vi "Script Edit Module Name.vi"(8 "error in":errorcluster, 10 "Library":refnum<class "Library.lvclass">, 11 "Project":refnum<class "Project.lvclass">) -> (0 "error out":errorcluster)   [LabVIEW 2020, in "Panther Dashboard.lvlib"]
uses:
  Panther Dashboard.lvlib
  Class/Library/Library.lvclass
  C:/GitClones/PantherDashboard/src/LabVIEW/Panther Dashboard/Class/LabVIEWItem/LabVIEWItem.lvclass
  Class/Project/Project.lvclass
  <vilib>/Utility/traverseref.llb/TRef TravTarget.ctl
  Class/Project/Project.lvclass/Project.ctl
  Class/LabVIEWItem/LabVIEWItem.lvclass/LabVIEWItem.ctl
  Class/Project/Read Main App Inst Ref.vi
  Class/LabVIEWItem/Read Item Path.vi
  <vilib>/Utility/traverseref.llb/VI Scripting - Traverse.lvlib
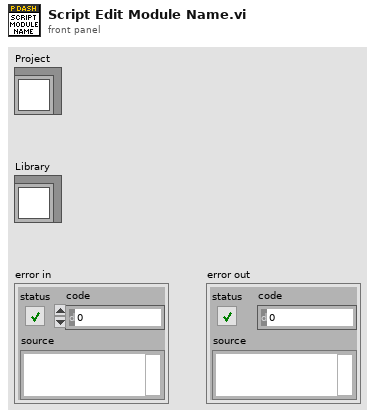
[diagram p1: front panel]
types:
  T1 = typedef "TRef TravTarget.ctl" = enum16{"FP", "BD", "Other"}
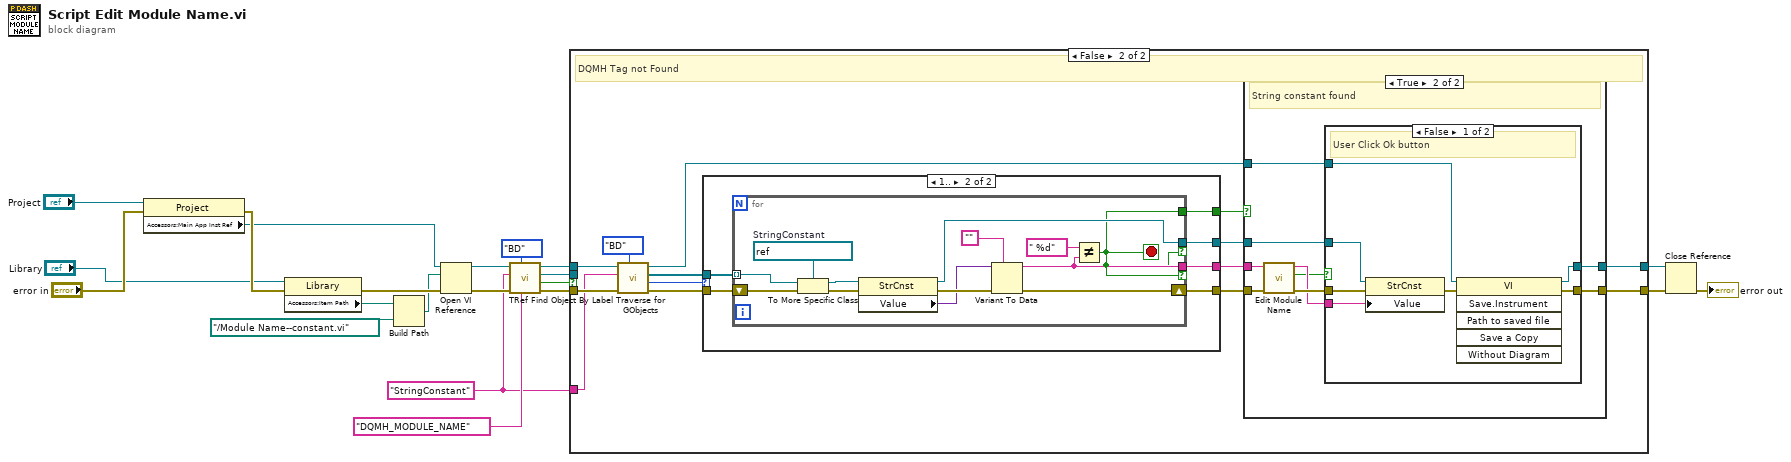
[diagram p0: block diagram]
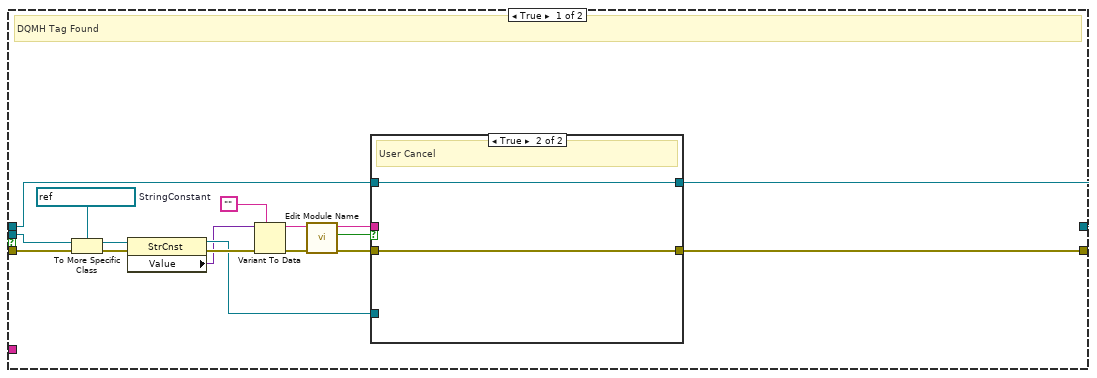
[diagram p2: hidden frame]
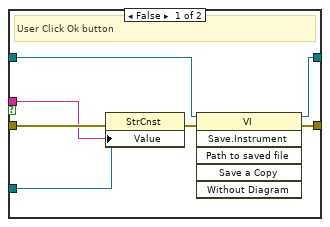
[diagram p3: hidden frame]
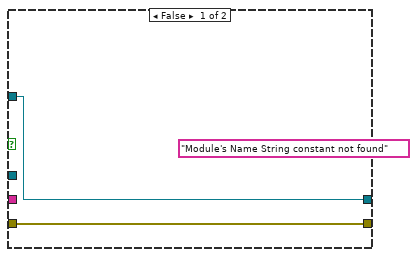
[diagram p4: hidden frame]
diagram:
  w4 = "StringConstant" ("Class Name")
  n1 = property class="Project"(reference="Project", error in="error in") -> (error out=w15:errorcluster, "Accessors:Main App Inst Ref"=w1:refnum<vi>)  [unwired: 1 out]
  n2 = property class="Library"(reference="Library", error in=w15) -> (error out=w21:errorcluster, "Accessors:Item Path"=w14:path)  [unwired: 1 out]
  n3 = Build Path(base path=w14, name or relative path=path "../Module Name--constant.vi") -> (appended path=w12:path)
  n4 = Open VI Reference(application reference (local)=w1, vi path=w12, error in (no error)=w21) -> (vi reference=w11:refnum<vi>, error out=w20:errorcluster)  [unwired: 3 in]
  n5 = call <vilib>:"TRef Find Object By Label.vi"("Label"="DQMH_MODULE_NAME", "Traverse Target"=TRef_TravTarget."BD", "error in (no error)"=w20, "Class Name"=w4, "VI Ref"=w11) -> ("error out"=w19:errorcluster, "Found?"=w8:bool, "Found Obj Ref"=w9:refnum<vi>, "dup VI Ref"=w6:refnum<vi>)  [unwired: 3 in]
  n6 = case shown="False" w8 {
    tunnel: w19 -> [w38 w59]
    tunnel: w9 -> [w32 _]
    tunnel: w6 -> [w26 w53]
    tunnel: [w25 w57] -> w5
    tunnel: [w34 w61] -> w17
    tunnel: w4 -> [_ w52]
    frame True {
      w31 = refnum<vi> refnum  # StringConstant
      # "DQMH Tag Found"
      n7 = To More Specific Class(target class=w31, reference=w32, error in=w38) -> (specific class reference=w30:refnum<vi>, error out=w37:errorcluster)
      n8 = property class="StrCnst"(reference=w30, error in=w37) -> (reference out=w29:refnum<vi>, error out=w36:errorcluster, "Value"=w24:variant)
      n9 = Variant To Data(error in=w36, type="", Variant=w24) -> (data=w22:string, error out=w33:errorcluster)
      n10 = call "Edit Module Name.vi"("error in"=w33, "Module Name Read"=w22) -> ("error out"=w35:errorcluster, "Canceled"=w27:bool, "New Module Name"=w28:string)  [unwired: 7 in]
      n11 = case shown="True" w27 {
        tunnel: w35 -> [w45 w47]
        tunnel: w29 -> [w42 _]
        tunnel: w28 -> [w41 _]
        tunnel: w26 -> [w40 w46]
        tunnel: [w39 w46] -> w25
        tunnel: [w44 w47] -> w34
        frame False {
          # "User Click Ok button"
          n12 = property class="StrCnst"(reference=w42, error in=w45, "Value"=w41) -> (error out=w43:errorcluster)  [unwired: 1 out]
          n13 = invoke class="VI" method="Save.Instrument"(reference=w40, error in=w43) -> (reference out=w39:refnum<vi>, error out=w44:errorcluster)  [unwired: 4 in, 4 out]
        }
        frame True {
          # "User Cancel"
        }
      }
    }
    frame False {
      # "DQMH Tag not Found"
      n14 = call <vilib>:"Traverse for GObjects.vi"("Traverse Target"=TRef_TravTarget."BD", "error in (no error)"=w59, "Class Name"=w52, "VI Refnum"=w53) -> ("error out"=w60:errorcluster, "# of Refs"=w55:i32, "References"=w54:refnum<vi>[], "dup VI Refnum"=w49:refnum<vi>)  [unwired: 4 in]
      n15 = case shown="1.." w55 {
        tunnel: w60 -> [w84 w90]
        tunnel: w54 -> [_ w88]
        tunnel: [w84 w89] -> w58
        tunnel: [FALSE w86] -> w50
        tunnel: [_ w87] -> w51
        tunnel: [_ w85] -> w48
        frame Default {
        }
        frame 1.. {
          n16 = for {
            tunnel: w88 -> [w97] mode=indexing
            shift-right: [w100] -> w89
            shift-left: w90 -> [w102]
            tunnel: [w96] -> w87 if=w91
            tunnel: [w91] -> w86
            tunnel: [w92] -> w85 if=w91
            stop <- w91 stop-if-true
            w98 = refnum<vi> refnum  # StringConstant
            n17 = To More Specific Class(target class=w98, reference=w97, error in=w102) -> (specific class reference=w99:refnum<vi>, error out=w103:errorcluster)
            n18 = property class="StrCnst"(reference=w99, error in=w103) -> (reference out=w96:refnum<vi>, error out=w101:errorcluster, "Value"=w93:variant)
            n19 = Variant To Data(error in=w101, type="", Variant=w93) -> (data=w92:string, error out=w100:errorcluster)
            n20 = Not Equal?(x=" %d" ("Append module ID to \nModule Name"), y=w92) -> (x != y?=w91:bool)
          }
        }
      }
      n21 = case shown="True" w50 {
        tunnel: [w64 w72] -> w61
        tunnel: [w63 w68] -> w57
        tunnel: w49 -> [w63 w67]
        tunnel: w58 -> [w64 w71]
        tunnel: w51 -> [_ w66]
        tunnel: w48 -> [_ w65]
        frame False {
          n22 = call "Status Updated.vi"("Status"="Module's Name String constant not found") -> ()  [unwired: 10 in, 1 out]
        }
        frame True {
          # "String constant found"
          n23 = call "Edit Module Name.vi"("error in"=w71, "Module Name Read"=w65) -> ("error out"=w73:errorcluster, "Canceled"=w69:bool, "New Module Name"=w70:string)  [unwired: 7 in]
          n24 = case shown="False" w69 {
            tunnel: w73 -> [w80 w82]
            tunnel: w70 -> [w77 _]
            tunnel: w67 -> [w76 w81]
            tunnel: [w75 w81] -> w68
            tunnel: [w79 w82] -> w72
            tunnel: w66 -> [w74 _]
            frame False {
              # "User Click Ok button"
              n25 = property class="StrCnst"(reference=w74, error in=w80, "Value"=w77) -> (error out=w78:errorcluster)  [unwired: 1 out]
              n26 = invoke class="VI" method="Save.Instrument"(reference=w76, error in=w78) -> (reference out=w75:refnum<vi>, error out=w79:errorcluster)  [unwired: 4 in, 4 out]
            }
            frame True {
              # "User Cancel"
            }
          }
        }
      }
    }
  }
  n27 = Close Reference(reference=w5, error in (no error)=w17) -> (error out=→"error out":errorcluster)
